vi "ReplaceSelfClosingStructureElements.vi"(11 "String In":string) -> (3 "String Out":string)   [LabVIEW 2017]
uses:
  <vilib>/regexp/Match Regular Expression.xnode
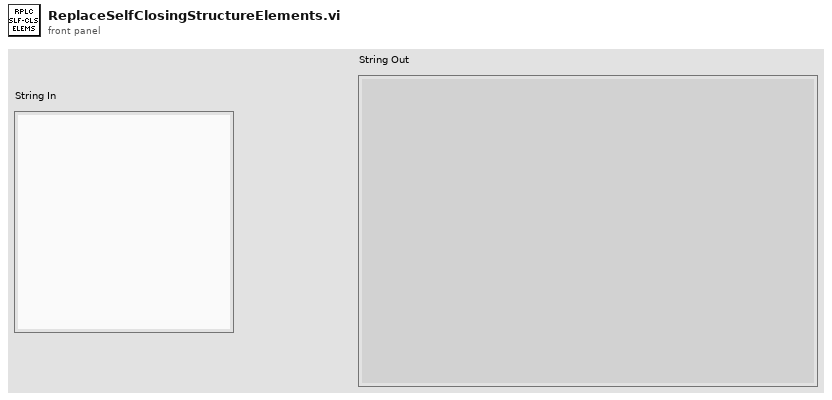
[diagram p1: front panel]
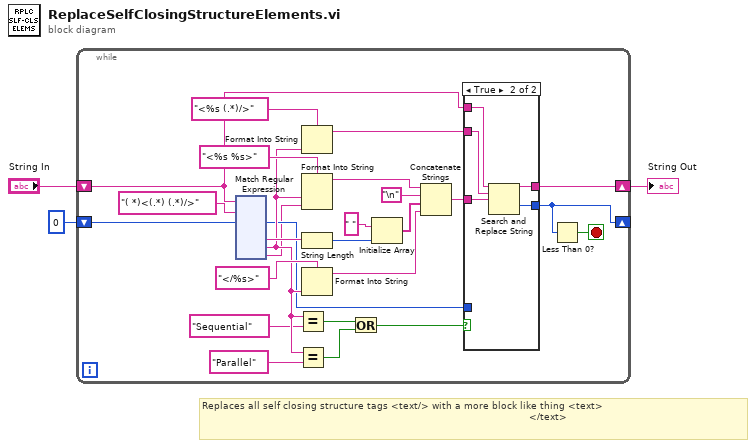
[diagram p0: block diagram]
diagram:
  # "Replaces all self closing structure tags <text/> with a more block like thing <text>\n                                                                                                             </text>"
  n1 = while {
    shift-right: [w29] -> w1
    shift-left: "String In" -> [w27]
    shift-right: [w24] -> _
    shift-left: 0 -> [w26]
    stop <- w28 stop-if-true
    n2 = xnode "Match Regular Expression"("input string"=w27, "regular expression"="( *)<(.*) (.*)/>" ("format string"), "offset (0)"=w26) -> ("offset past match"=w5:i32, "submatch 1"=w25:string, "submatch 2"=w13:string, "submatch 3"=w4:string)  [unwired: 3 in, 4 out]
    n3 = Equal?(x=w13, y="Sequential") -> (x = y?=w10:bool)
    n4 = Equal?(x=w13, y="Parallel") -> (x = y?=w9:bool)
    n5 = Format Into String(format string="<%s (.*)/>" ("search string"), w13) -> (resulting string=w8:string)  [unwired: 2 in, 1 out]
    n6 = Format Into String(format string="<%s %s>" ("replace string (\"\")"), w13, w4) -> (resulting string=w19:string)  [unwired: 2 in, 1 out]
    n7 = String Length(string=w25) -> (length=w14:i32)
    n8 = Format Into String(format string="</%s>" ("replace string (\"\")"), w13) -> (resulting string=w16:string)  [unwired: 2 in, 1 out]
    n9 = Or(x=w10, y=w9) -> (x .or. y?=w6:bool)
    n10 = Initialize Array(" " ("search string"), w14) -> (w22:string[])
    n11 = Concatenate Strings(w19, "\n", w22, w16) -> (w7:string)
    n12 = case shown="True" w6 {
      tunnel: [w31 w36] -> w29
      tunnel: w27 -> [w31 w35]
      tunnel: [w30 w34] -> w24
      tunnel: w8 -> [_ w33]
      tunnel: w7 -> [_ w32]
      tunnel: w5 -> [w30 _]
      frame False {
      }
      frame True {
        n13 = Search and Replace String(input string=w35, search string=w33, replace string=w32) -> (result string=w36:string, offset past replacement=w34:i32)  [unwired: 5 in, 2 out]
      }
    }
    n14 = Less Than 0?(x=w24) -> (x < 0?=w28:bool)
  }
  "String Out" <- w1
